vi "Build High Priority Message Configuration.vi"(6 "Group":i32, 7 "Virtual Memory Unit in":refnum<class "Virtual Memory Unit.lvclass">, 8 "error in (no error)":errorcluster, 10 "Starting Address":u16 format="%04x", 11 "Major Frame in":refnum<class "Major Frame.lvclass">) -> (0 "error out":errorcluster, 2 "Next Available Address":u16 format="%04x", 3 "Major Frame out":refnum<class "Major Frame.lvclass">, 5 "Virtual Memory Unit out":refnum<class "Virtual Memory Unit.lvclass">)   [LabVIEW 2020, in "BCI-1553 API.lvlib" / "Major Frame.lvclass"]
doc: "Generates some basic config info for the HP async control words.\n\nThe actual asynchronous msg will fill in the remainder of the details as necessary."
uses:
  Major Frame.lvclass
  Dependencies/Virtual Memory Unit/Virtual Memory Unit.lvclass
  Major Frame.lvclass/Major Frame.ctl
  BCI-1553 API.lvlib
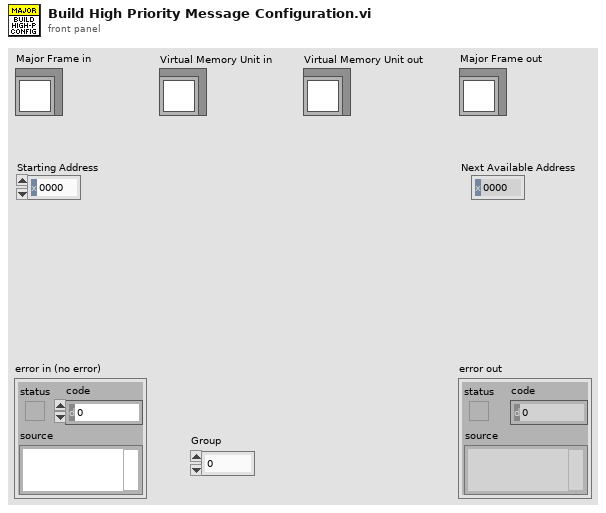
[diagram p1: front panel]
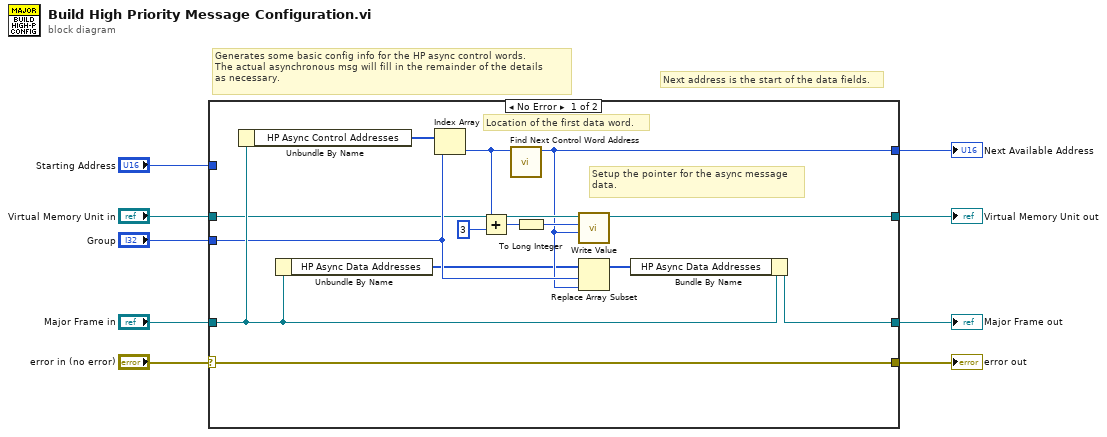
[diagram p0: block diagram]
diagram:
  # "Next address is the start of the data fields."
  # "Generates some basic config info for the HP async control words.\nThe actual asynchronous msg will fill in the remainder of the details\nas necessary."
  n1 = case shown="No Error" "error in (no error)" {
    selector: "error in (no error)" -> [w20 w25]
    tunnel: [w20 w25] -> w8
    tunnel: [w21 w24] -> w7
    tunnel: "Major Frame in" -> [w22 w24]
    tunnel: "Virtual Memory Unit in" -> [w18 _]
    tunnel: [w17 _] -> w2
    tunnel: "Starting Address" -> [_ _]
    tunnel: [w12 _] -> w1
    tunnel: "Group" -> [w19 _]
    frame No Error {
      # "Setup the pointer for the async message\ndata."
      # "Location of the first data word."
      n2 = Unbundle By Name(w22) -> ("HP Async Control Addresses"=w23:u16[])
      n3 = Unbundle By Name(w22) -> ("HP Async Data Addresses"=w11:u16[])
      n4 = Index Array(array=w23, index=w19) -> (element=w16:u16)
      n5 = Add(x=w16, y=u16 3) -> (x+y=w14:u16)
      n6 = call "Find Next Control Word Address.vi"("Starting Address"=w16) -> ("0xHHHX Address"=w12:u16)  [unwired: 10 in]
      n7 = To Long Integer(number=w14) -> (32bit integer=w13:i32)
      n8 = call "Write Value.vi"("Value"=w12, "Index"=w13, "Virtual Memory Unit in"=w18) -> ("Virtual Memory Unit out"=w17:refnum<class "Virtual Memory Unit.lvclass">)  [unwired: 7 in, 1 out]
      n9 = Replace Array Subset(array=w11, new element=w12, index=w19) -> (w10:u16[])
      n10 = Bundle By Name(cluster=w22, "HP Async Data Addresses"=w10) -> (w21:refnum<class "Major Frame.lvclass">)
    }
    frame Error {
    }
  }
  "error out" <- w8
  "Major Frame out" <- w7
  "Virtual Memory Unit out" <- w2
  "Next Available Address" <- w1
